vi "Read Configuration Class Name.vi"(8 "error in (no error)":errorcluster, 11 "Targets in":refnum<class "Targets.lvclass">) -> (0 "error out":errorcluster, 2 "Configuration Class Name":string[](array[string]), 3 "Targets out":refnum<class "Targets.lvclass">)   [LabVIEW 2013, in "PL Framework Configuration Tool.lvlib" / "Targets.lvclass"]
uses:
  Targets.lvclass
  Targets.lvclass/Targets.ctl
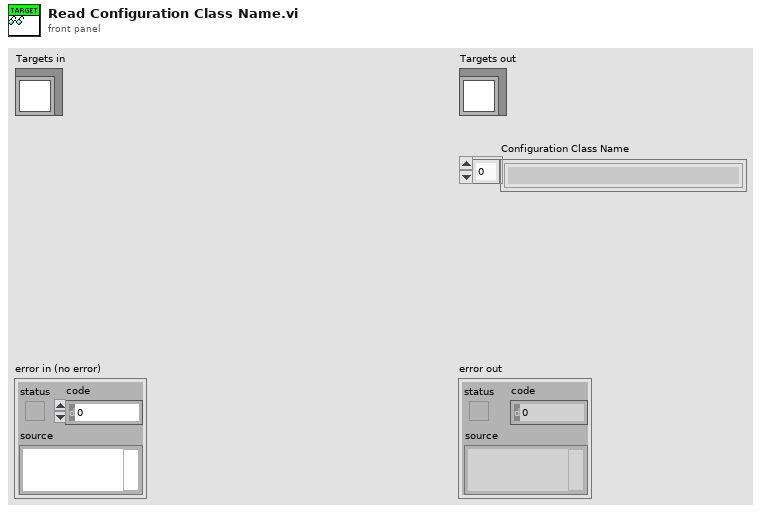
[diagram p1: front panel]
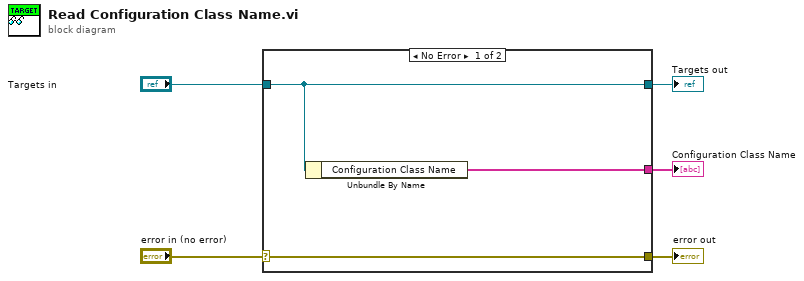
[diagram p0: block diagram]
diagram:
  n1 = case shown="No Error" "error in (no error)" {
    selector: "error in (no error)" -> [w8 w9]
    tunnel: [w8 w9] -> w4
    tunnel: [w7 w10] -> w2
    tunnel: "Targets in" -> [w7 w10]
    tunnel: [w6 _] -> w1
    frame No Error {
      n2 = Unbundle By Name(w7) -> ("Configuration Class Name"=w6:string[])
    }
    frame Error {
    }
  }
  "error out" <- w4
  "Targets out" <- w2
  "Configuration Class Name" <- w1
